vi "ESP32_Task_4.vi"() -> ()   [LabVIEW 2022 SP3]
doc: "This example performs writes and reads on a serial port, as directed by the user. You can press the Write and Read buttons, and change the Read Count, while the example is running.\n\nThe parameters set for the serial port must match the parameters of the connected instrument or device. In this example, the Read Count parameter specifies the number of bytes that the serial port reads. If there were more bytes at the port than the specified number, those bytes would not be read. If there were less bytes at the port than the specified number, you would receive a timeout error.\n\nThis example expands upon the flow control options for XON and XOFF, allowing the user to choose those control characters. Also, the user can enable or disable a termination character. Some devices require a termination character in order to identify the end of command strings. Some devices send a termination character to signify the end of data to be read. This example shows how you can end the Read operation once a termination character is detected in the buffer and/or append a termination character at the end of the Write data."
uses:
  Serial - Settings.ctl
  Serial - XON-XOFF Characters.ctl
  Serial - ASCII Characters.ctl
  ESP32-PSOC-State Machine.ctl
  <vilib>/Instr/_visa.llb/VISA Flush IO Buffer Mask.ctl
  <vilib>/Instr/_visa.llb/VISA Configure Serial Port (Instr).vi
panel:
  out "concatenated string":string
  in  "Numeric":dbl
  out "number 2":dbl
  out "number":dbl
  out "String":string
  in  "Difficulty":T1
  out "error":bool
  out "Connected":bool
  out "Serial Settings:Number of Bytes at Serial Port":u32
  out "Response 2":string
  in  "Toggle LED":bool
  in  "Enum":T2
  in  "Termination Character":u8=10 format="%.0x"
  in  "End Write on Termination Character?":bool=TRUE
  in  "Stop":bool
  out "Read Count":u32=1000
  out "Response":string
  in  "XON/XOFF Characters":T3={"XON"=enum."DC1", "XOFF"=enum."DC3"}
  in  "Serial Settings":T5={"baud rate"=115200, "data bits"=8, "parity"=enum."None", "stop bits"=10, "flow control"=0} {"flow control" items=["None"=0, "XON/XOFF"=1, "RTS/CTS"=2, "DTR/DSR"=4]; "stop bits" items=["1.0"=10, "1.5"=15, "2.0"=20]; "data bits" min=5 max=8 step=1; "baud rate" items=["75"=75, "110"=110, "134"=134, "150"=150, "300"=300, "600"=600, "1200"=1200, "1800"=1800, "2400"=2400, "4800"=4800, "7200"=7200, "9600"=9600, "14400"=14400, "19200"=19200, "28800"=28800, "38400"=38400, "56000"=56000, "57600"=57600, "115200"=115200, "128000"=128000, "230400"=230400]}
  in  "End Read on Termination Character?":bool=TRUE
  in  "VISA resource name":refnum<visa-resource-name>="COM4"
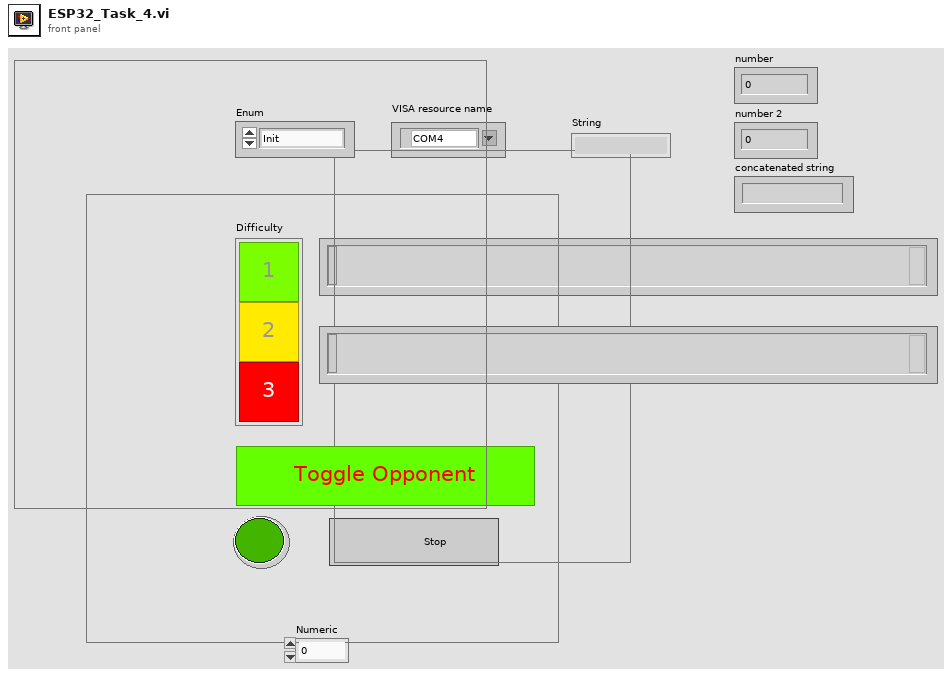
[diagram p1: front panel]
types:
  T1 = cluster{"Command A":bool, "Command B":bool, "Command C":bool}
  T2 = typedef "ESP32-PSOC-State Machine.ctl" = enum8{"Init", "Connect", "idle", "send", "wait", "receive", "que", "error", "exit"}
  T3 = typedef "Serial - XON-XOFF Characters.ctl" = cluster{"XON":T4, "XOFF":T4}
  T4 = typedef "Serial - ASCII Characters.ctl" = enum16{"NUL", "SOH", "STX", "ETX", "EOT", "ENQ", "ACK", "BEL", "BS", "HT", "LF", "VT", "FF", "CR", "SO", "SI", "DLE", "DC1", "DC2", "DC3", "DC4", "NAK", "SYN", "ETB", "CAN", "EM", "SUB", "ESC", "FS", "GS", "RS", "US", "SP", "!", "\"", "#", "$", "%", "&", "'", "(", ")", "*", "+", ",", "- (-)", ".", "/", "0", "1", "2", "3", "4", "5", "6", "7", "8", "9", ":", ";", "<", "=", ">", "?", "@", "A", "B", "C", "D", "E", "F", "G", "H", "I", "J", "K", "L", "M", "N", "O", "P", "Q", "R", "S", "T", "U", "V", "W", "X", "Y", "Z", "[", "\\", "]", "^", "_", "`", "a", "b", "c", "d", "e", "f", "g", "h", "i", "j", "k", "l", "m", "n", "o", "p", "q", "r", "s", "t", "u", "v", "w", "x", "y", "z", "{", "|", "}", "~"}
  T5 = typedef "Serial - Settings.ctl" = cluster{"baud rate":u32, "data bits":u16, "parity":enum16{"None", "Odd", "Even", "Mark", "Space"}, "stop bits":u16, "flow control":u16}
  T6 = typedef "VISA Flush IO Buffer Mask.ctl" = u16
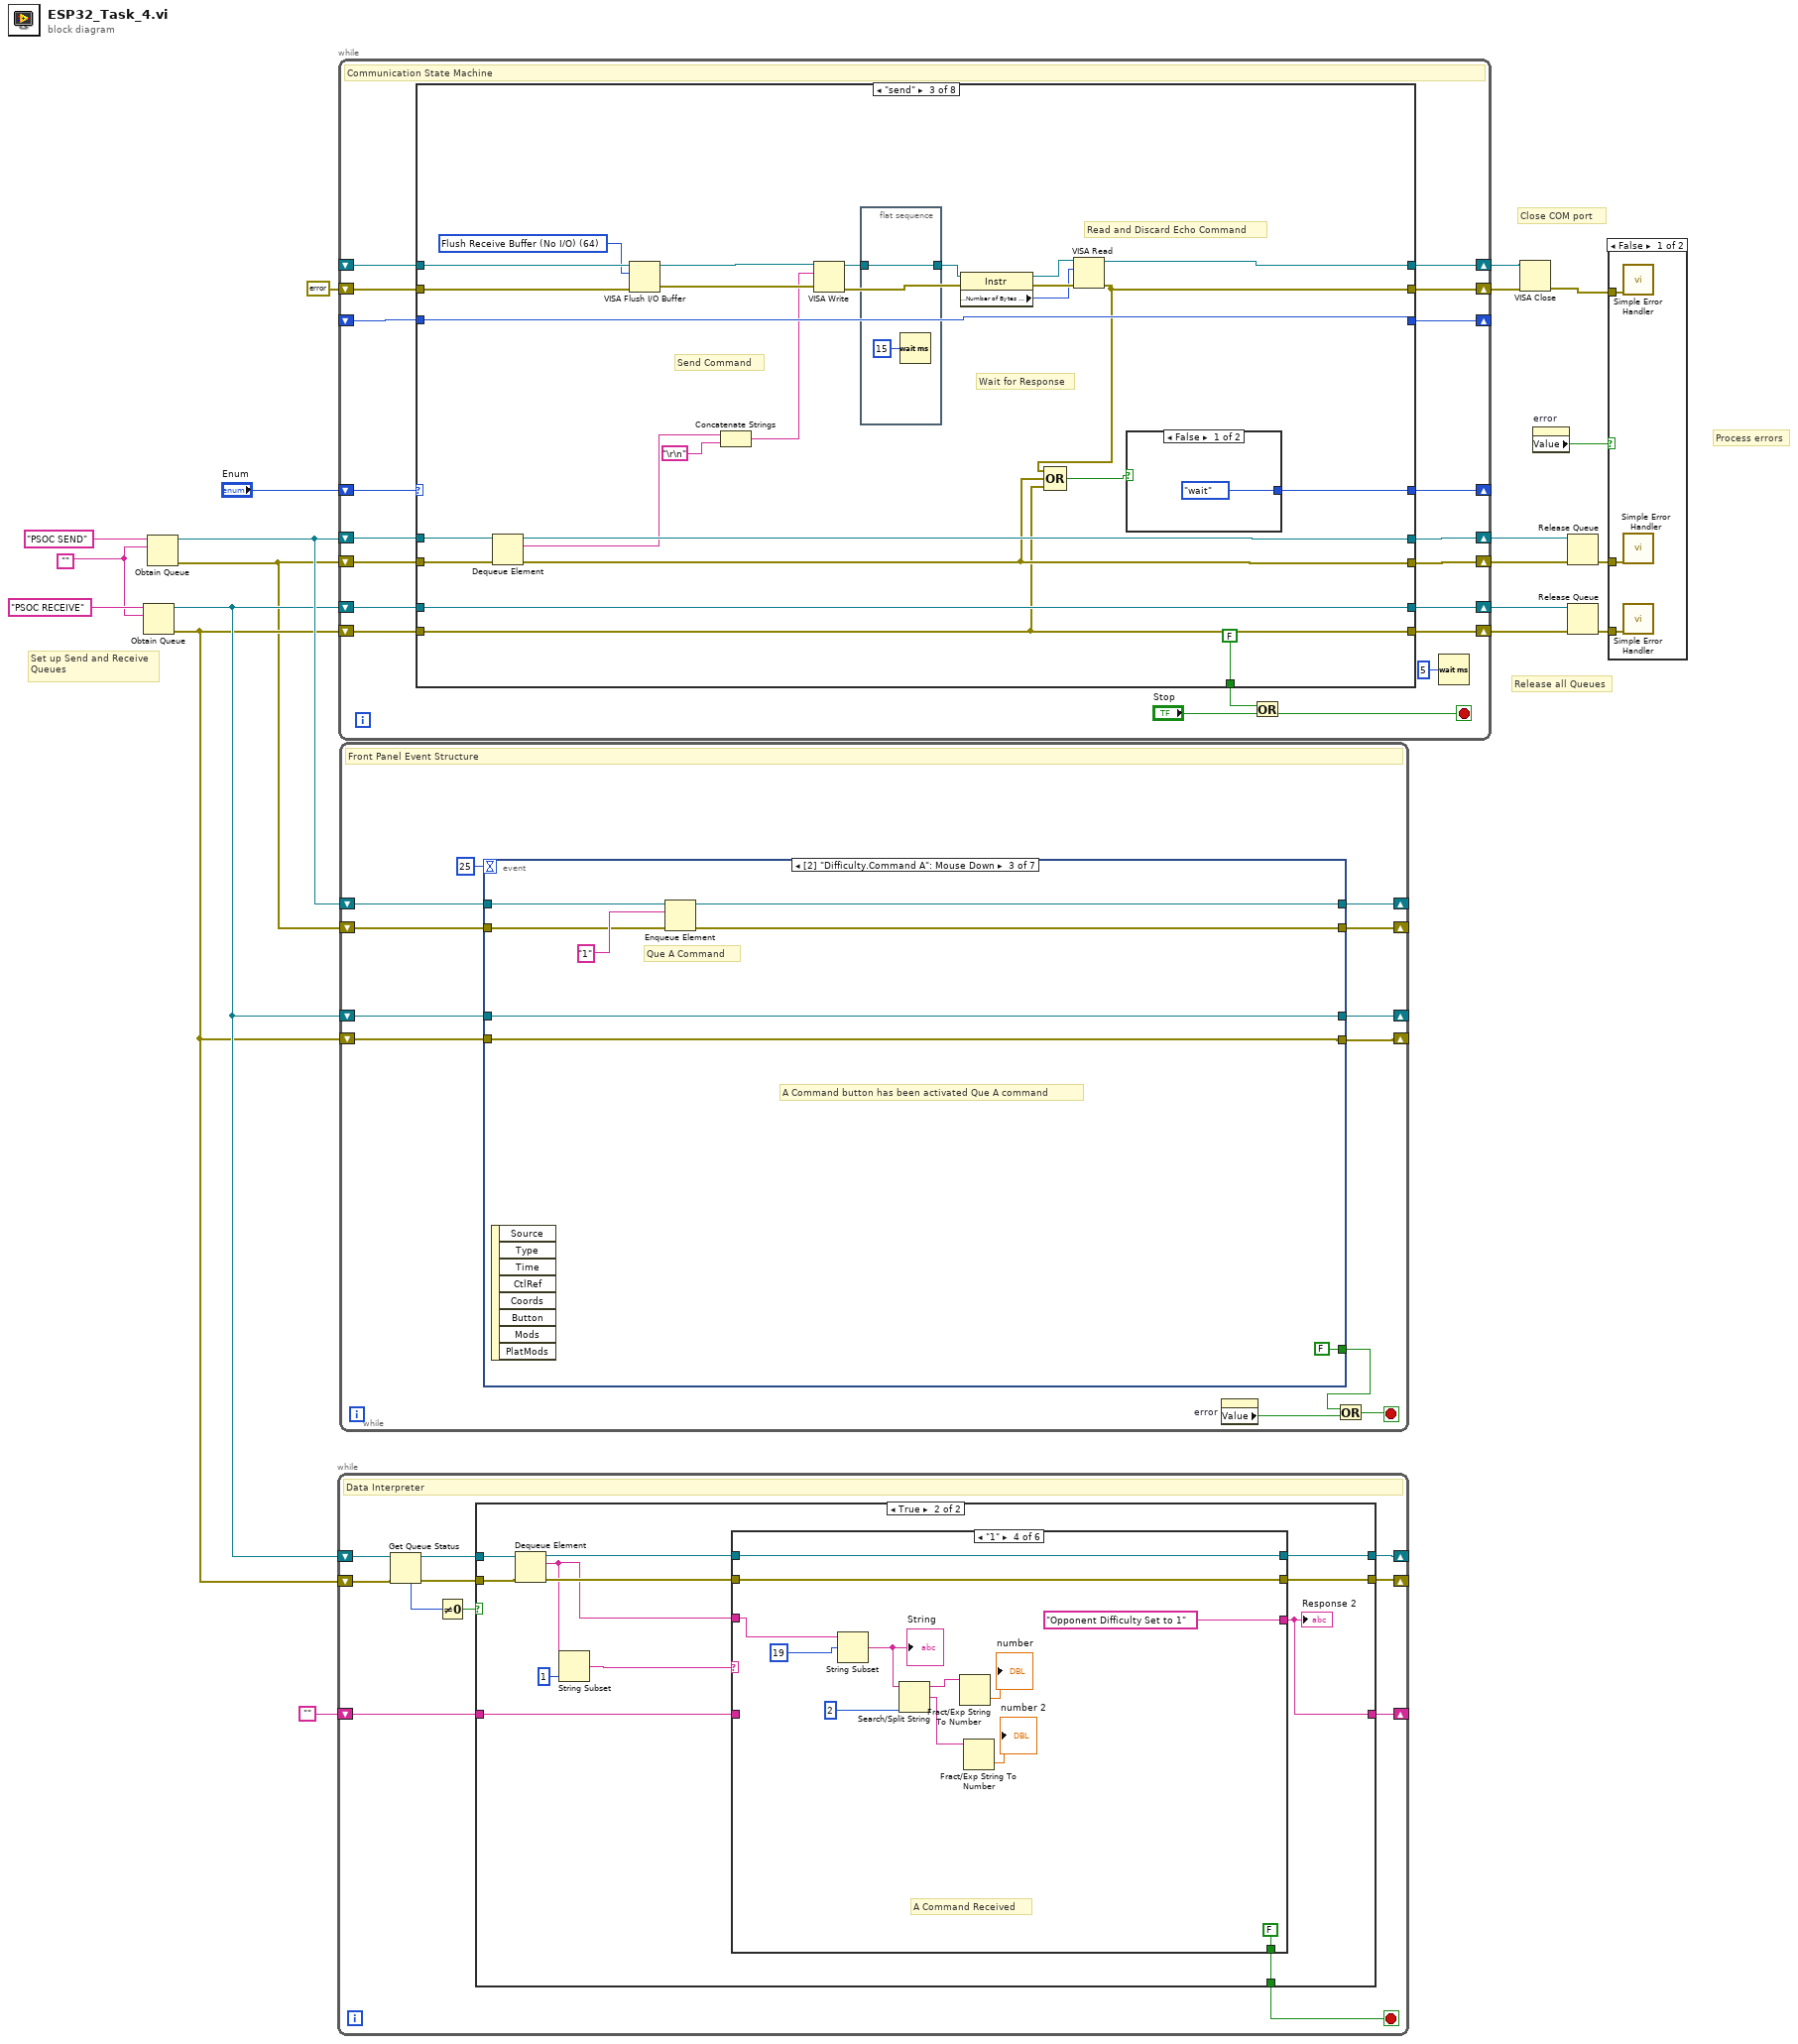
[diagram p0: block diagram]
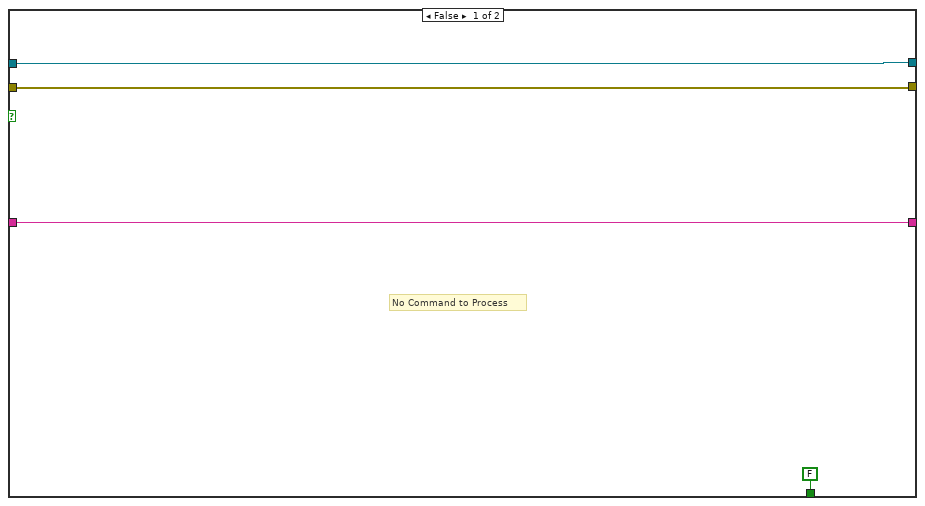
[diagram p3: hidden frame]
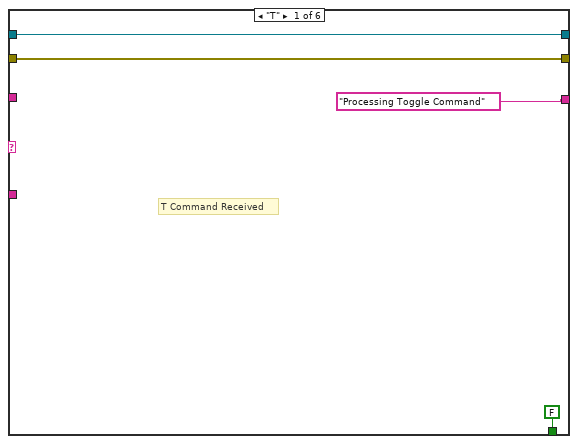
[diagram p4: hidden frame]
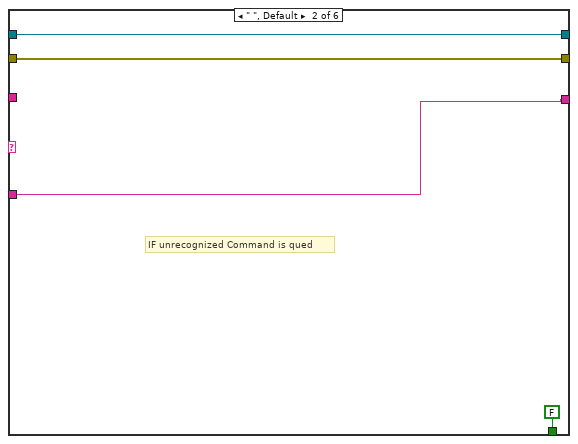
[diagram p5: hidden frame]
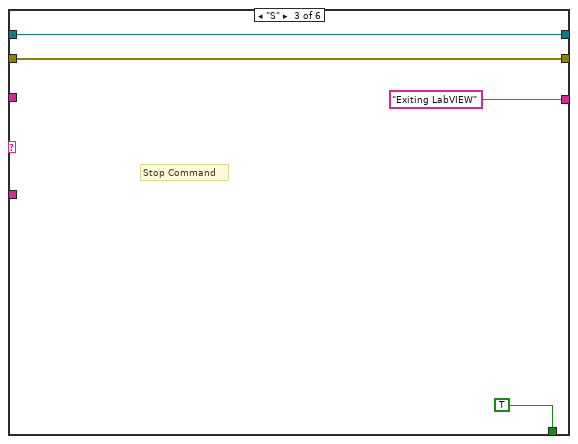
[diagram p6: hidden frame]
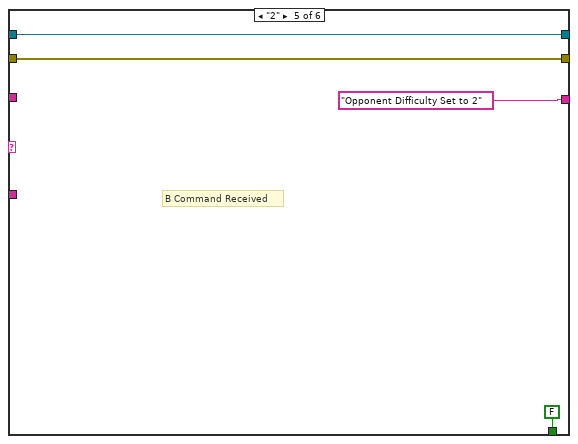
[diagram p7: hidden frame]
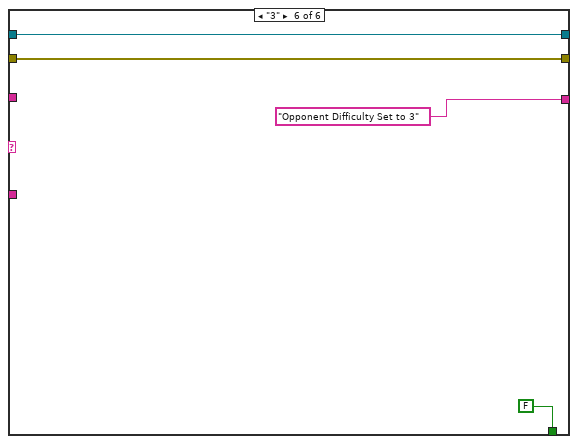
[diagram p8: hidden frame]
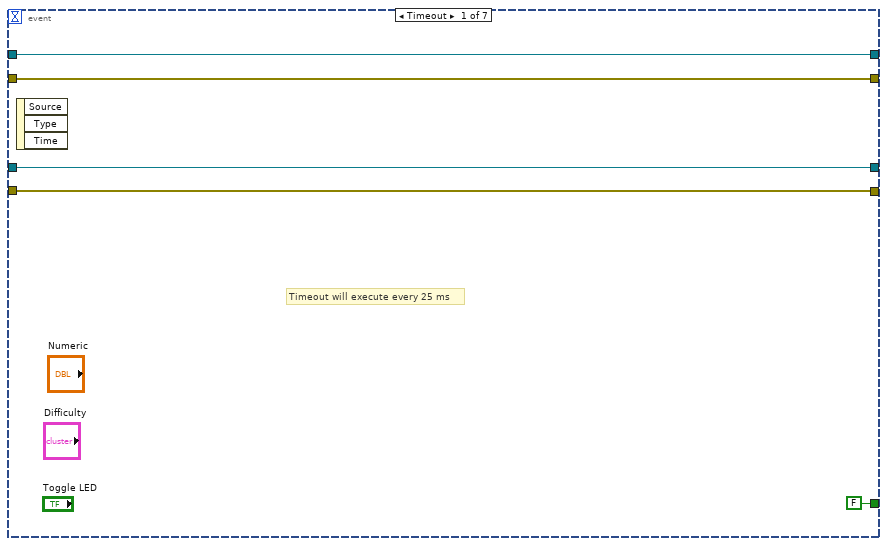
[diagram p9: hidden frame]
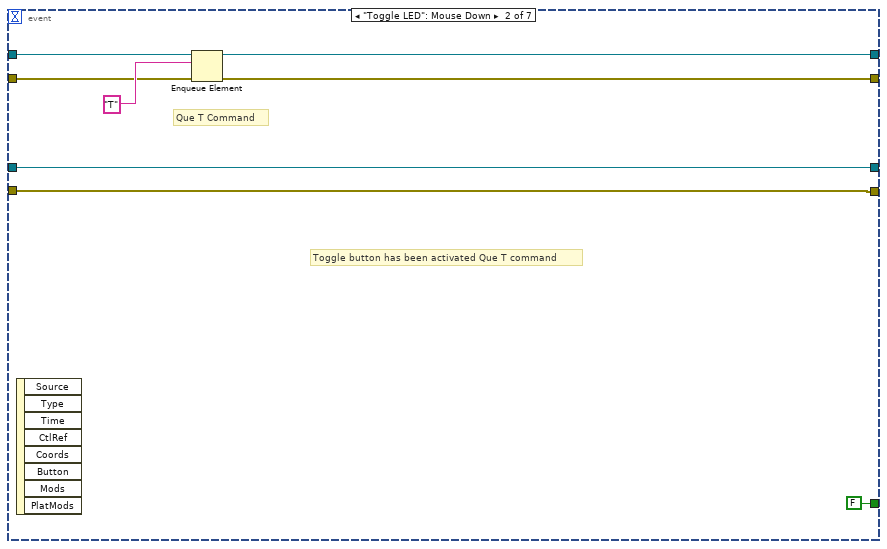
[diagram p10: hidden frame]
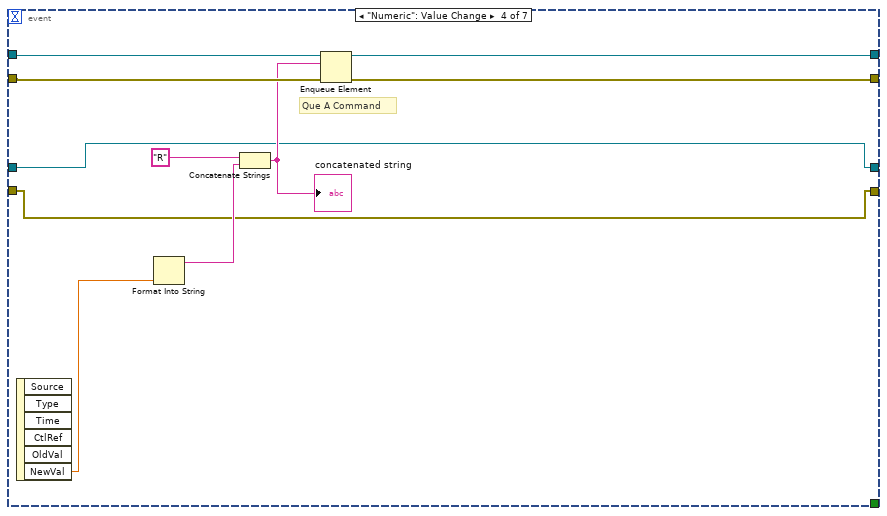
[diagram p11: hidden frame]
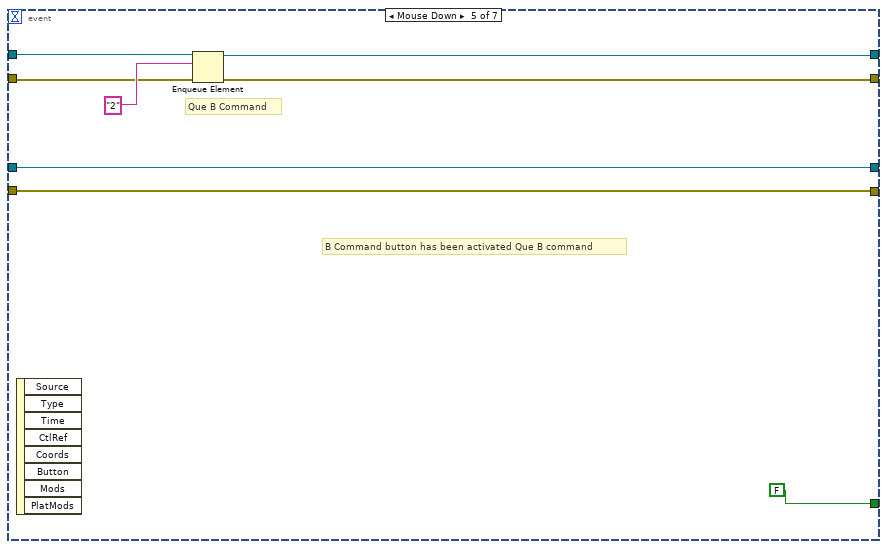
[diagram p12: hidden frame]
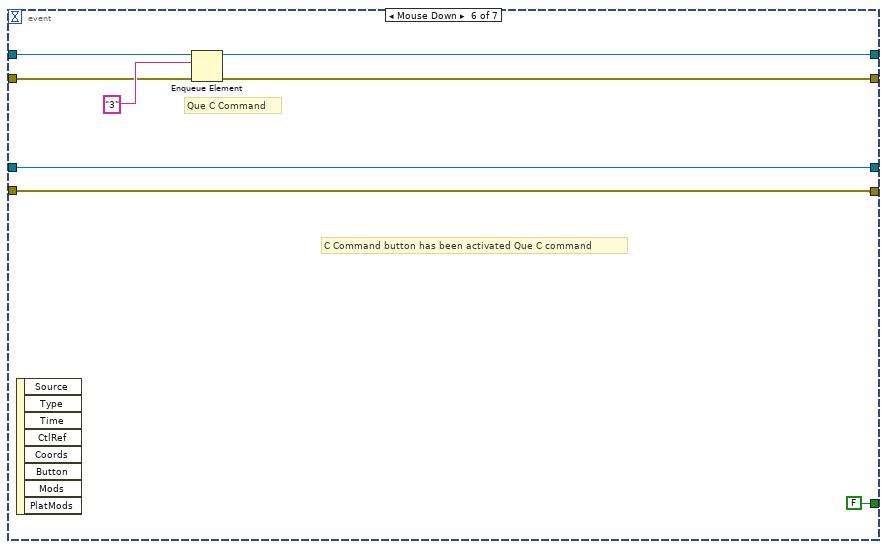
[diagram p13: hidden frame]
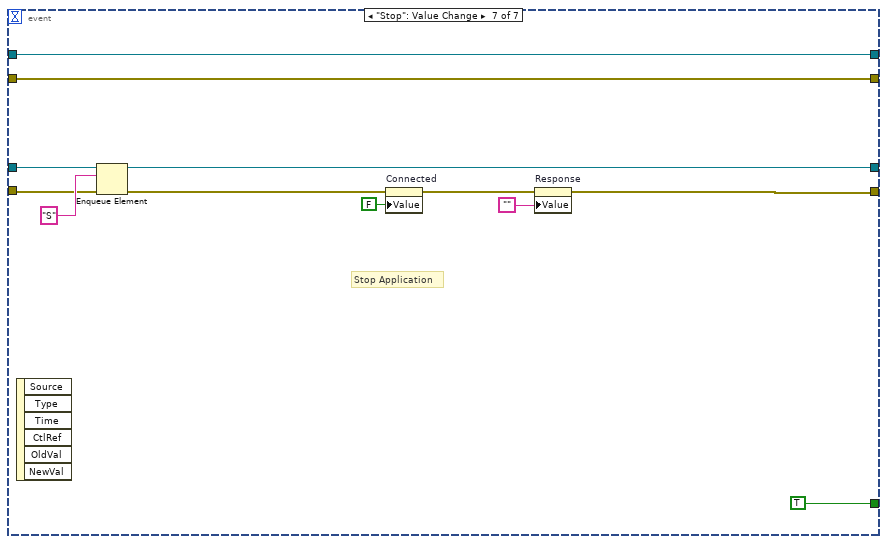
[diagram p14: hidden frame]
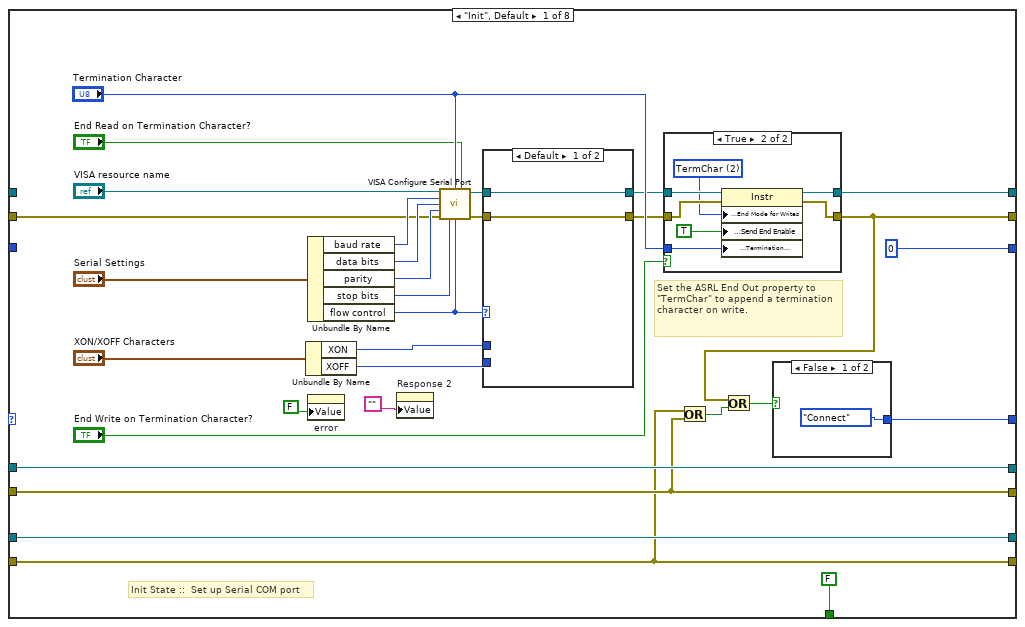
[diagram p15: hidden frame]
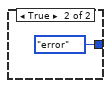
[diagram p16: hidden frame]
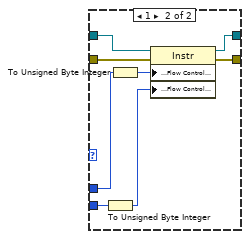
[diagram p18: hidden frame]
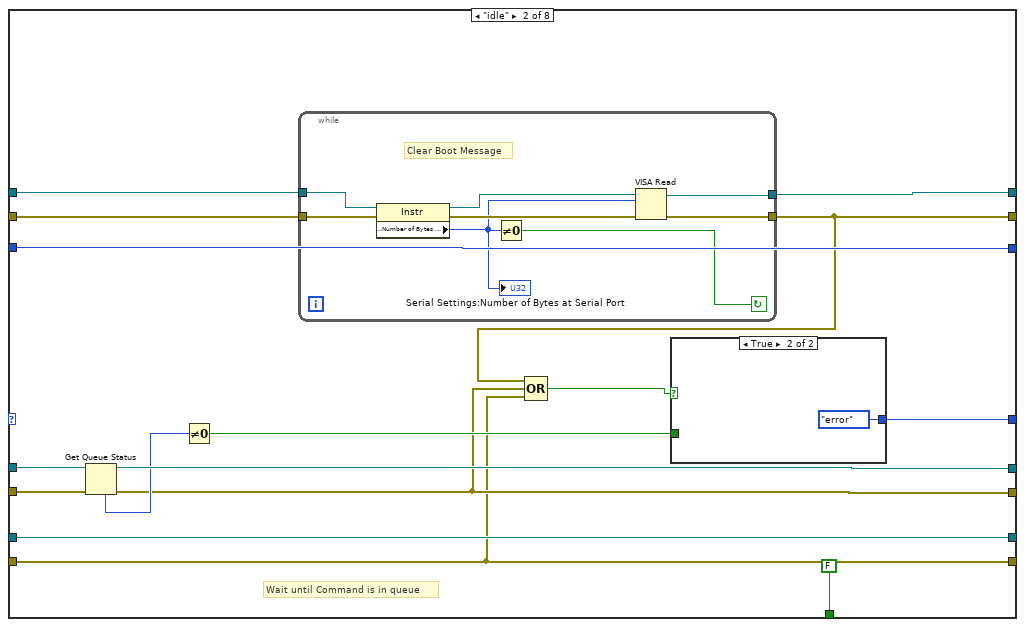
[diagram p19: hidden frame]
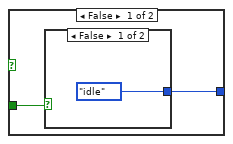
[diagram p20: hidden frame]
diagram:
  w10 = ""
  # "Process errors"
  # "Release all Queues"
  # "Close COM port"
  # "Set up Send and Receive\nQueues"
  n1 = Obtain Queue(name (unnamed)="PSOC RECEIVE", element data type=w10) -> (queue out=w9:refnum<queue>, error out=w8:errorcluster)  [unwired: 3 in, 1 out]
  n2 = Obtain Queue(name (unnamed)="PSOC SEND", element data type=w10) -> (queue out=w12:refnum<queue>, error out=w2:errorcluster)  [unwired: 3 in, 1 out]
  n3 = while {
    shift-right: [w25] -> _
    shift-left: w9 -> [w31]
    shift-right: [w24] -> _
    shift-left: w8 -> [w30]
    shift-right: [w22] -> _
    shift-left: "" -> [w21]
    stop <- w23 stop-if-true
    # "Data Interpreter"
    n4 = Get Queue Status(queue=w31, error in (no error)=w30) -> (queue out=w27:refnum<queue>, error out=w26:errorcluster, # elements in queue=w29:i32)  [unwired: 1 in, 5 out]
    n5 = Not Equal To 0?(x=w29) -> (x != 0?=w28:bool)
    n6 = case shown="True" w28 {
      tunnel: w27 -> [w35 w47]
      tunnel: w26 -> [w34 w40]
      tunnel: [w35 w45] -> w25
      tunnel: [w34 w44] -> w24
      tunnel: [FALSE w43] -> w23
      tunnel: [w32 w42] -> w22
      tunnel: w21 -> [w32 w41]
      frame False {
        # "No Command to Process"
      }
      frame True {
        n7 = Dequeue Element(queue=w47, error in (no error)=w40) -> (queue out=w38:refnum<queue>, element=w37:string, error out=w39:errorcluster)  [unwired: 1 in, 1 out]
        n8 = String Subset(string=w37, length (rest)=1 ("length (rest)")) -> (substring=w36:string)  [unwired: 1 in]
        n9 = case shown="\"1\"" w36 {
          tunnel: w38 -> [w51 w55 w59 w68 w75 w78]
          tunnel: w39 -> [w50 w54 w58 w71 w74 w77]
          tunnel: [w51 w55 w59 w68 w75 w78] -> w45
          tunnel: [w50 w54 w58 w71 w74 w77] -> w44
          tunnel: w37 -> [_ _ _ w67 _ _]
          tunnel: [FALSE FALSE TRUE FALSE FALSE FALSE] -> w43
          tunnel: ["Processing Toggle Command" w52 "Exiting LabVIEW" "Opponent Difficulty Set to 1" "Opponent Difficulty Set to 2" "Opponent Difficulty Set to 3"] -> w42
          tunnel: w41 -> [_ w52 _ _ _ _]
          frame "T" {
            # "T Command Received"
          }
          frame " ", Default {
            # "IF unrecognized Command is qued"
          }
          frame "S" {
            # "Stop Command"
          }
          frame "1" {
            # "A Command Received"
            n10 = String Subset(string=w67, offset (0)=19 ("length (rest)")) -> (substring=w64:string)  [unwired: 1 in]
            "String" <- w64
            n11 = Search/Split String(string=w64, offset (0)=2 ("length (rest)")) -> (substring before match=w60:string, match + rest of string=w61:string)  [unwired: 1 in, 1 out]
            n12 = Fract/Exp String To Number(string=w60) -> (number=→"number":dbl)  [unwired: 3 in, 1 out]
            n13 = Fract/Exp String To Number(string=w61) -> (number=→"number 2":dbl)  [unwired: 3 in, 1 out]
          }
          frame "2" {
            # "B Command Received"
          }
          frame "3" {
          }
        }
        "Response 2" <- w42
      }
    }
  }
  n14 = while {
    shift-right: [w91] -> w20
    shift-left: w12 -> [w99]
    shift-right: [w90] -> w18
    shift-left: w2 -> [w98]
    shift-right: [w89] -> w19
    shift-left: w9 -> [w97]
    shift-right: [w88] -> w15
    shift-left: w8 -> [w96]
    shift-right: [w83] -> _
    shift-left: "Enum" -> [w82]
    shift-right: [w95] -> w14
    shift-left: _ -> [w92]
    shift-right: [w94] -> w13
    shift-left: errorcluster {"status"=FALSE, "code"=0, "source"=""} ("error out") -> [w93]
    shift-right: [w87] -> _
    shift-left: _ -> [w86]
    stop <- w81 stop-if-true
    # "Communication State Machine"
    n15 = case shown="\"send\"" w82 {
      selector: w82 -> [_ _ _ _ _ _ w301 _]
      tunnel: [w129 w165 w204 w221 w258 w285 w300 w323] -> w91
      tunnel: [w103 w155 w195 w215 w240 w282 w299 w322] -> w90
      tunnel: [w109 w163 w196 w224 w259 ESP32-PSOC-State_Machine."exit" ("Enum") w301 ESP32-PSOC-State_Machine."idle" ("Enum")] -> w83
      tunnel: w99 -> [w129 w167 w206 w221 w258 w285 w300 w323]
      tunnel: w98 -> [w103 w166 w205 w215 w240 w282 w299 w322]
      tunnel: w97 -> [w130 w161 w203 w218 w253 w284 w298 w321]
      tunnel: w96 -> [w102 w154 w194 w214 w239 w281 w289 w320]
      tunnel: [w111 w158 w190 w223 w248 w287 w304 w325] -> w95
      tunnel: [w105 w156 w191 w216 w241 w283 w303 w326] -> w94
      tunnel: w93 -> [w107 w157 w199 w222 w243 w283 w303 w327]
      tunnel: w92 -> [_ w159 w201 w212 w256 w287 w304 w328]
      tunnel: [w130 w161 w203 w218 w251 w284 w296 w321] -> w89
      tunnel: [w102 w154 w194 w214 w252 w281 w292 w320] -> w88
      tunnel: [u32 0 ("Bytes at Port") w160 w202 w220 w254 w286 w302 w324] -> w87
      tunnel: w86 -> [_ w160 w202 _ w250 w286 w302 w324]
      tunnel: [FALSE FALSE FALSE FALSE FALSE FALSE TRUE FALSE] -> w80
      frame "Init", Default {
        # "Init State ::  Set up Serial COM port"
        # "Set the ASRL End Out property to \"TermChar\" to append a termination character on write."
        n16 = Unbundle By Name("XON/XOFF Characters") -> ("XON"=w123:T4, "XOFF"=w124:T4)
        n17 = Unbundle By Name("Serial Settings") -> ("baud rate"=w119:u32, "data bits"=w118:u16, "parity"=w117:enum16{"None", "Odd", "Even", "Mark", "Space"}, "stop bits"=w116:u16, "flow control"=w122:u16)
        n18 = property on="error" class="Bool (strict)"("Value"=FALSE ("error")) -> ()  [unwired: 2 in, 2 out]
        n19 = property on="Response 2" class="Str"("Value"="") -> ()  [unwired: 2 in, 2 out]
        n20 = call-poly "VISA Configure Serial Port"("VISA resource name"="VISA resource name", "termination char\n(0xA = '\\n' = LF)"="Termination Character", "Enable Termination\nChar (T)"="End Read on Termination Character?", "baud rate (9600)"=w119, "data bits (8)"=w118, "parity (0:none)"=w117, "error in (no error)"=w107, "stop bits (10: 1 bit)"=w116, "flow control (0:none)"=w122) -> ("VISA resource name out"=w115:refnum<visa-resource-name>, "error out"=w114:errorcluster)  [unwired: 1 in, 4 out]
        n21 = case shown="Default" w122 {
          tunnel: [w142 w151] -> w125
          tunnel: [w143 w150] -> w126
          tunnel: w114 -> [w142 w149]
          tunnel: w115 -> [w143 w148]
          tunnel: w123 -> [_ w147]
          tunnel: w124 -> [_ w146]
          frame Default {
          }
          frame 1 {
            n22 = To Unsigned Byte Integer(number=w146) -> (unsigned 8bit integer=w145:u8)
            n23 = To Unsigned Byte Integer(number=w147) -> (unsigned 8bit integer=w144:u8)
            n24 = property class="Instr"(reference=w148, error in=w149, "Serial Settings:Flow Control XON Character"=w144, "Serial Settings:Flow Control XOFF Character"=w145) -> (reference out=w150:refnum<visa-resource-name>, error out=w151:errorcluster)
          }
        }
        n25 = case shown="True" "End Write on Termination Character?" {
          tunnel: w126 -> [w133 w141]
          tunnel: w125 -> [w134 w140]
          tunnel: [w133 w139] -> w111
          tunnel: [w134 w138] -> w105
          tunnel: "Termination Character" -> [_ w136]
          frame False {
          }
          frame True {
            w137 = u16 2 items=["None", "LastBit", "TermChar", "Break"] ("Serial Settings:Serial End Mode for Writes")
            n26 = property class="Instr"(reference=w141, error in=w140, "Serial Settings:End Mode for Writes"=w137, "Message Based Settings:Send End Enable"=TRUE, "Message Based Settings:Termination Character"=w136) -> (reference out=w139:refnum<visa-resource-name>, error out=w138:errorcluster)
          }
        }
        n27 = Or(x=w102, y=w103) -> (x .or. y?=w104:bool)
        n28 = Or(x=w105, y=w104) -> (x .or. y?=w106:bool)
        n29 = case shown="False" w106 {
          tunnel: [ESP32-PSOC-State_Machine."Connect" ("Enum") ESP32-PSOC-State_Machine."error" ("Enum")] -> w109
          frame False {
          }
          frame True {
          }
        }
      }
      frame "idle" {
        # "Wait until Command is in queue"
        n30 = Get Queue Status(queue=w167, error in (no error)=w166) -> (queue out=w165:refnum<queue>, error out=w155:errorcluster, # elements in queue=w164:i32)  [unwired: 1 in, 5 out]
        n31 = Not Equal To 0?(x=w164) -> (x != 0?=w162:bool)
        n32 = while {
          tunnel: w159 -> [w180]
          tunnel: [w176] -> w158
          tunnel: w157 -> [w179]
          tunnel: [w174] -> w156
          stop <- w178 continue-if-true
          # "Clear Boot Message"
          n33 = property class="Instr"(reference=w180, error in=w179) -> (reference out=w177:refnum<visa-resource-name>, error out=w175:errorcluster, "Serial Settings:Number of Bytes at Serial Port"=w173:u32)
          "Serial Settings:Number of Bytes at Serial Port" <- w173
          n34 = Not Equal To 0?(x=w173) -> (x != 0?=w178:bool)
          n35 = VISA Read(VISA resource name=w177, byte count=w173, error in (no error)=w175) -> (VISA resource name out=w176:refnum<visa-resource-name>, error out=w174:errorcluster)  [unwired: 2 out]
        }
        n36 = Compound Arithmetic op=OR(w156, w155, w154) -> (w153:bool)
        n37 = case shown="True" w153 {
          tunnel: [w169 ESP32-PSOC-State_Machine."error" ("Enum")] -> w163
          tunnel: w162 -> [w168 _]
          frame False {
            n38 = case shown="False" w168 {
              tunnel: [ESP32-PSOC-State_Machine."idle" ("Enum") ESP32-PSOC-State_Machine."send" ("Enum")] -> w169
              frame False {
              }
              frame True {
              }
            }
          }
          frame True {
          }
        }
      }
      frame "send" {
        w197 = T6 64 items=["Flush Receive Buffer"=16, "Write Transmit Buffer to Device"=32, "Flush Receive Buffer (No I/O)"=64, "Flush Transmit Buffer"=128] ("Mask")
        # "Read and Discard Echo Command"
        # "Wait for Response"
        # "Send Command"
        n39 = Dequeue Element(queue=w206, error in (no error)=w205) -> (queue out=w204:refnum<queue>, element=w184:string, error out=w195:errorcluster)  [unwired: 1 in, 1 out]
        n40 = VISA Flush I/O Buffer(VISA resource name=w201, mask (16)=w197, error in (no error)=w199) -> (VISA resource name out=w200:refnum<visa-resource-name>, error out=w198:errorcluster)
        n41 = Concatenate Strings(w184, "\r\n") -> (w183:string)
        n42 = VISA Write(VISA resource name=w200, write buffer=w183, error in (no error)=w198) -> (VISA resource name out=w182:refnum<visa-resource-name>, error out=w188:errorcluster)  [unwired: 1 out]
        n43 = flat-sequence {
          tunnel: w182 -> [w208]
          tunnel: [w208] -> w181
          frame #0 {
            n44 = Wait (ms)(milliseconds to wait=u32 15) -> ()  [unwired: 1 out]
          }
        }
        n45 = property class="Instr"(reference=w181, error in=w188) -> (reference out=w189:refnum<visa-resource-name>, error out=w187:errorcluster, "Serial Settings:Number of Bytes at Serial Port"=w186:u32)
        n46 = VISA Read(VISA resource name=w189, byte count=w186, error in (no error)=w187) -> (VISA resource name out=w190:refnum<visa-resource-name>, error out=w191:errorcluster)  [unwired: 2 out]
        n47 = Compound Arithmetic op=OR(w191, w195, w194) -> (w193:bool)
        n48 = case shown="False" w193 {
          tunnel: [ESP32-PSOC-State_Machine."wait" ("Enum") ESP32-PSOC-State_Machine."error" ("Enum")] -> w196
          frame False {
          }
          frame True {
          }
        }
      }
      frame "wait" {
        # "Wait for actual Response"
        n49 = flat-sequence {
          tunnel: w212 -> [w226]
          tunnel: [w226] -> w211
          frame #0 {
            n50 = Wait (ms)(milliseconds to wait=u32 15) -> ()  [unwired: 1 out]
          }
        }
        n51 = property class="Instr"(reference=w211, error in=w222) -> (reference out=w223:refnum<visa-resource-name>, error out=w216:errorcluster, "Serial Settings:Number of Bytes at Serial Port"=w220:u32)
        n52 = Not Equal To 0?(x=w220) -> (x != 0?=w219:bool)
        n53 = Compound Arithmetic op=OR(w216, w215, w214) -> (w217:bool)
        n54 = case shown="False" w217 {
          tunnel: [w228 ESP32-PSOC-State_Machine."error" ("Enum")] -> w224
          tunnel: w219 -> [w227 _]
          frame False {
            n55 = case shown="True" w227 {
              tunnel: [ESP32-PSOC-State_Machine."wait" ("Enum") ESP32-PSOC-State_Machine."receive" ("Enum")] -> w228
              frame False {
              }
              frame True {
              }
            }
          }
          frame True {
          }
        }
      }
      frame "receive" {
        # "Process Response and Display"
        # "Read Response"
        n56 = VISA Read(VISA resource name=w256, byte count=w250, error in (no error)=w243) -> (VISA resource name out=w249:refnum<visa-resource-name>, read buffer=w245:string, error out=w255:errorcluster)  [unwired: 1 out]
        n57 = String To Byte Array(string=w245) -> (unsigned byte array=w244:u8[])
        n58 = property class="Instr"(reference=w249, error in=w255) -> (reference out=w248:refnum<visa-resource-name>, error out=w242:errorcluster, "Serial Settings:Number of Bytes at Serial Port"=w254:u32)
        n59 = Index Array(array=w244, index=0) -> (element=w236:u8)
        n60 = Equal?(x=w236, y=u8 13) -> (x = y?=w234:bool)
        n61 = Equal?(x=w236, y=u8 10) -> (x = y?=w233:bool)
        n62 = Not Or(1:w233, 2:w234) -> (0:w232:bool)
        n63 = Not Equal To 0?(x=w254) -> (x != 0?=w257:bool)
        n64 = case shown="True" w232 {
          tunnel: w244 -> [_ w276]
          tunnel: w242 -> [w265 w270]
          tunnel: [w265 w269] -> w241
          frame False {
          }
          frame True {
            n65 = Delete From Array(array=w276, length=1, index=0) -> (array with subset deleted=w273:u8[])  [unwired: 1 out]
            n66 = Byte Array To String(unsigned byte array=w273) -> (string=w268:string)
            n67 = property on="Response" class="Str"(error in=w270, "Value"="") -> (error out=w271:errorcluster)  [unwired: 1 in, 1 out]
            n68 = String Subset(string=w268, length (rest)=17 ("length")) -> (substring=w267:string)  [unwired: 1 in]
            n69 = property on="Response" class="Str"(error in=w271, "Value"=w267) -> (error out=w269:errorcluster)  [unwired: 1 in, 1 out]
          }
        }
        n70 = Compound Arithmetic op=OR(w241, w240, w239) -> (w238:bool)
        n71 = Enqueue Element(queue=w253, element=w245, error in (no error)=w239) -> (queue out=w251:refnum<queue>, error out=w252:errorcluster)  [unwired: 1 in, 1 out]
        n72 = case shown="False" w238 {
          tunnel: [w261 ESP32-PSOC-State_Machine."error" ("Enum")] -> w259
          tunnel: w257 -> [w260 _]
          frame False {
            n73 = case shown="False" w260 {
              tunnel: [ESP32-PSOC-State_Machine."idle" ("Enum") ESP32-PSOC-State_Machine."receive" ("Enum")] -> w261
              frame False {
              }
              frame True {
              }
            }
          }
          frame True {
          }
        }
        "Read Count" <- w250
      }
      frame "error" {
        # "Process any error"
        n74 = Build Array(w283, w282, w281) -> (w280:errorcluster[])
        n75 = for {
          tunnel: w280 -> [w288] mode=indexing
          n76 = call <vilib>:"General Error Handler.vi"("error in (no error)"=w288) -> ()  [unwired: 10 in, 5 out]
        }
        "error" <- TRUE ("error")
      }
      frame "exit" {
        # "Exit due to error"
        n77 = Enqueue Element(queue=w298, element="S", error in (no error)=w289) -> (queue out=w296:refnum<queue>, error out=w294:errorcluster)  [unwired: 1 in, 1 out]
        n78 = property on="Connected" class="Bool (strict)"(error in=w294, "Value"=FALSE ("Connected")) -> (error out=w293:errorcluster)  [unwired: 1 in, 1 out]
        n79 = property on="Response" class="Str"(error in=w293, "Value"="") -> (error out=w292:errorcluster)  [unwired: 1 in, 1 out]
      }
      frame "Connect" {
        # "Validating connection"
        # "Send ID to validate connection"
        # "Clear any residual characters"
        n80 = while {
          shift-right: [w352] -> w316
          shift-left: w327 -> [w358]
          shift-right: [w351] -> w317
          shift-left: w328 -> [w357]
          stop <- w356 continue-if-true
          n81 = property class="Instr"(reference=w357, error in=w358) -> (reference out=w354:refnum<visa-resource-name>, error out=w353:errorcluster, "Bytes at Port"=w350:u32)
          n82 = VISA Read(VISA resource name=w354, byte count=w350, error in (no error)=w353) -> (VISA resource name out=w351:refnum<visa-resource-name>, read buffer=w349:string, error out=w352:errorcluster)  [unwired: 1 out]
          n83 = Wait (ms)(milliseconds to wait=u32 5) -> ()  [unwired: 1 out]
          n84 = Search/Split String(string=w349, search string/char (-)="Commands") -> (match + rest of string=w347:string)  [unwired: 1 in, 2 out]
          n85 = String Length(string=w347) -> (length=w346:i32)
          n86 = Equal To 0?(x=w346) -> (x = 0?=w356:bool)
        }
        n87 = Concatenate Strings("I" ("write buffer"), "\r\n") -> (w305:string)
        n88 = VISA Write(VISA resource name=w317, write buffer=w305, error in (no error)=w316) -> (VISA resource name out=w311:refnum<visa-resource-name>, error out=w315:errorcluster)  [unwired: 1 out]
        n89 = flat-sequence {
          tunnel: w311 -> [w345]
          tunnel: [w345] -> w310
          frame #0 {
            n90 = Wait (ms)(milliseconds to wait=u32 5) -> ()  [unwired: 1 out]
          }
        }
        n91 = property class="Instr"(reference=w310, error in=w315) -> (reference out=w313:refnum<visa-resource-name>, error out=w314:errorcluster, "Bytes at Port"=w312:u32)
        n92 = VISA Read(VISA resource name=w313, byte count=w312, error in (no error)=w314) -> (VISA resource name out=w308:refnum<visa-resource-name>, error out=w309:errorcluster)  [unwired: 2 out]
        n93 = while {
          shift-right: [w332] -> w326
          shift-left: w309 -> [w338]
          shift-right: [w333] -> w325
          shift-left: w308 -> [w331]
          stop <- w329 stop-if-true
          n94 = flat-sequence {
            tunnel: w331 -> [w343]
            tunnel: [w343] -> w330
            frame #0 {
              n95 = Wait (ms)(milliseconds to wait=u32 15) -> ()  [unwired: 1 out]
            }
          }
          n96 = property class="Instr"(reference=w330, error in=w338) -> (reference out=w336:refnum<visa-resource-name>, error out=w337:errorcluster, "Bytes at Port"=w335:u32)
          n97 = VISA Read(VISA resource name=w336, byte count=w335, error in (no error)=w337) -> (VISA resource name out=w333:refnum<visa-resource-name>, read buffer=w334:string, error out=w332:errorcluster)  [unwired: 1 out]
          n98 = Search/Split String(string=w334, search string/char (-)="IESP32") -> (match + rest of string=w340:string)  [unwired: 1 in, 2 out]
          n99 = String Length(string=w340) -> (length=w339:i32)
          n100 = Not Equal To 0?(x=w339) -> (x != 0?=w329:bool)
          "Connected" <- w329
        }
      }
    }
    n101 = Or(x=w80, y="Stop") -> (x .or. y?=w81:bool)
    n102 = Wait (ms)(milliseconds to wait=u32 5) -> ()  [unwired: 1 out]
  }
  n103 = while {
    shift-right: [w367] -> _
    shift-left: w12 -> [w368]
    shift-right: [w366] -> _
    shift-left: w2 -> [w369]
    shift-right: [w362] -> _
    shift-left: w9 -> [w365]
    shift-right: [w363] -> _
    shift-left: w8 -> [w364]
    stop <- w359 stop-if-true
    # "Front Panel Event Structure"
    n104 = event shown="[2] \"Difficulty.Command A\": Mouse Down" {
      selector: _ -> [_ _ _ _ _ _ _]
      dyn-events: _ -> [_ _ _ _ _ _ _]
      timeout: 25 -> [_ _ _ _ _ _ _]
      tunnel: w369 -> [w373 w381 w389 w400 w405 w415 w427]
      tunnel: w368 -> [w374 w383 w391 w401 w406 w417 w428]
      tunnel: [w374 w380 w388 w399 w408 w414 w428] -> w367
      tunnel: [w373 w379 w387 w398 w407 w413 w427] -> w366
      tunnel: [FALSE FALSE FALSE _ FALSE FALSE TRUE] -> w361
      tunnel: w365 -> [w372 w377 w385 w393 w404 w411 w426]
      tunnel: w364 -> [w371 w376 w384 w392 w403 w410 w424]
      tunnel: [w371 w376 w384 w392 w403 w410 w419] -> w363
      tunnel: [w372 w377 w385 w393 w404 w411 w423] -> w362
      event Timeout {
        # "Timeout will execute every 25 ms"
        n105 = event-data() -> ()  [unwired: 1 in, 3 out]
      }
      event "Toggle LED": Mouse Down {
        # "Que T Command"
        # "Toggle button has been activated Que T command"
        n106 = event-data() -> ()  [unwired: 1 in, 8 out]
        n107 = Enqueue Element(queue=w383, element="T", error in (no error)=w381) -> (queue out=w380:refnum<queue>, error out=w379:errorcluster)  [unwired: 1 in, 1 out]
      }
      event "Difficulty.Command A": Mouse Down {
        # "Que A Command"
        # "A Command button has been activated Que A command"
        n108 = event-data() -> ()  [unwired: 1 in, 8 out]
        n109 = Enqueue Element(queue=w391, element="1", error in (no error)=w389) -> (queue out=w388:refnum<queue>, error out=w387:errorcluster)  [unwired: 1 in, 1 out]
      }
      event "Numeric": Value Change {
        # "Que A Command"
        n110 = event-data() -> ("NewVal"=w397:dbl)  [unwired: 1 in, 5 out]
        n111 = Format Into String(w397) -> (resulting string=w395:string)  [unwired: 3 in, 1 out]
        n112 = Concatenate Strings("R", w395) -> (w394:string)
        "concatenated string" <- w394
        n113 = Enqueue Element(queue=w401, element=w394, error in (no error)=w400) -> (queue out=w399:refnum<queue>, error out=w398:errorcluster)  [unwired: 1 in, 1 out]
      }
      event "Difficulty.Command B": Mouse Down {
        # "Que B Command"
        # "B Command button has been activated Que B command"
        n114 = event-data() -> ()  [unwired: 1 in, 8 out]
        n115 = Enqueue Element(queue=w406, element="2", error in (no error)=w405) -> (queue out=w408:refnum<queue>, error out=w407:errorcluster)  [unwired: 1 in, 1 out]
      }
      event "Difficulty.Command C": Mouse Down {
        # "Que C Command"
        # "C Command button has been activated Que C command"
        n116 = event-data() -> ()  [unwired: 1 in, 8 out]
        n117 = Enqueue Element(queue=w417, element="3", error in (no error)=w415) -> (queue out=w414:refnum<queue>, error out=w413:errorcluster)  [unwired: 1 in, 1 out]
      }
      event "Stop": Value Change {
        # "Stop Application"
        n118 = event-data() -> ()  [unwired: 1 in, 6 out]
        n119 = Enqueue Element(queue=w426, element="S", error in (no error)=w424) -> (queue out=w423:refnum<queue>, error out=w422:errorcluster)  [unwired: 1 in, 1 out]
        n120 = property on="Connected" class="Bool (strict)"(error in=w422, "Value"=FALSE ("Connected")) -> (error out=w420:errorcluster)  [unwired: 1 in, 1 out]
        n121 = property on="Response" class="Str"(error in=w420, "Value"="") -> (error out=w419:errorcluster)  [unwired: 1 in, 1 out]
      }
    }
    n122 = property on="error" class="Bool (strict)"() -> ("Value"=w360:bool)  [unwired: 2 in, 2 out]
    n123 = Or(x=w361, y=w360) -> (x .or. y?=w359:bool)
  }
  n124 = VISA Close(VISA resource name=w14, error in (no error)=w13) -> (error out=w5:errorcluster)
  n125 = property on="error" class="Bool (strict)"() -> ("Value"=w1:bool)  [unwired: 2 in, 2 out]
  n126 = Release Queue(queue=w20, error in (no error)=w18) -> (error out=w4:errorcluster)  [unwired: 1 in, 2 out]
  n127 = Release Queue(queue=w19, error in (no error)=w15) -> (error out=w3:errorcluster)  [unwired: 1 in, 2 out]
  n128 = case shown="False" w1 {
    tunnel: w5 -> [w432 _]
    tunnel: w4 -> [w431 _]
    tunnel: w3 -> [w430 _]
    frame False {
      n129 = call <vilib>:"Simple Error Handler.vi"("error in (no error)"=w432) -> ()  [unwired: 1 in, 8 out]
      n130 = call <vilib>:"Simple Error Handler.vi"("error in (no error)"=w431) -> ()  [unwired: 1 in, 8 out]
      n131 = call <vilib>:"Simple Error Handler.vi"("error in (no error)"=w430) -> ()  [unwired: 1 in, 8 out]
    }
    frame True {
    }
  }
